vi "Get Named Range (String).vi"(8 "error in":errorcluster, 10 "Named Range Identifier":string, 11 "SpreadsheetDocument":refnum<k24>) -> (0 "error out":errorcluster, 2 "Cells":string[][](array[string]), 3 "SpreadsheetDocument out":refnum<k24>)   [LabVIEW 2021, in "Open Xml.lvlib"]
uses:
  Open Xml.lvlib
  C:/Users/tupp_js/.nuget/packages/documentformat.openxml/3.3.0/lib/net46/DocumentFormat.OpenXml.dll
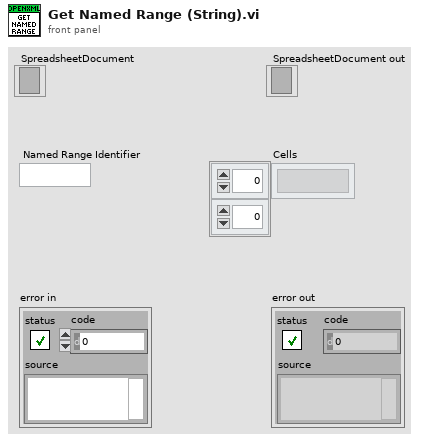
[diagram p1: front panel]
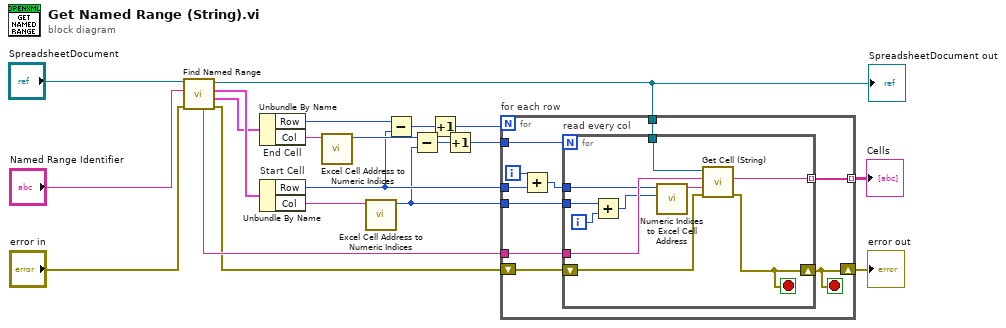
[diagram p0: block diagram]
diagram:
  n1 = call "Find Named Range.vi"("error in"="error in", "Range Identifier"="Named Range Identifier", "SpreadsheetDocument"="SpreadsheetDocument") -> ("error out"=w4:errorcluster, "End Cell"=w18:cluster{"Col":string, "Row":i32}, "Start Cell"=w19:cluster{"Col":string, "Row":i32}, "SpreadsheetDocument"=w1:refnum<k24>, "Sheet Name"=w6:string)  [unwired: 4 in]
  "SpreadsheetDocument out" <- w1
  n2 = Unbundle By Name "End Cell"(w18) -> ("Row"=w11:i32, "Col"=w16:string)
  n3 = Unbundle By Name "Start Cell"(w19) -> ("Row"=w8:i32, "Col"=w17:string)
  n4 = call "Excel Cell Address to Numeric Indices.vi"("Cell Name"=w16) -> ("Column Number"=w14:i32)  [unwired: 9 in, 1 out]
  n5 = call "Excel Cell Address to Numeric Indices.vi"("Cell Name"=w17) -> ("Column Number"=w7:i32)  [unwired: 9 in, 1 out]
  n6 = Subtract(x=w11, y=w8) -> (x-y=w10:i32)
  n7 = Subtract(x=w14, y=w7) -> (x-y=w12:i32)
  n8 = Increment(x=w10) -> (x+1=w9:i32)
  n9 = Increment(x=w12) -> (x+1=w13:i32)
  n10 = for "for each row" {
    N: w9 -> [_]
    tunnel: w13 -> [w30]
    tunnel: w8 -> [w26]
    tunnel: w1 -> [w29]
    tunnel: w7 -> [w28]
    tunnel: w6 -> [w27]
    tunnel: [w25] -> w5 mode=indexing
    shift-right: [w21] -> w3
    shift-left: w4 -> [w22]
    i -> [w23]
    stop <- w21 stop-if-true
    n11 = Add(x=w23, y=w26) -> (x+y=w24:i32)
    n12 = for "read every col" {
      N: w30 -> [_]
      tunnel: w29 -> [w40]
      tunnel: w28 -> [w37]
      tunnel: w27 -> [w39]
      tunnel: w24 -> [w36]
      tunnel: [w35] -> w25 mode=indexing
      shift-right: [w31] -> w21
      shift-left: w22 -> [w32]
      i -> [w33]
      stop <- w31 stop-if-true
      n13 = Add(x=w37, y=w33) -> (x+y=w34:i32)
      n14 = call "Numeric Indices to Excel Cell Address.vi"("Column"=w34, "Row"=w36) -> ("Cell Address"=w38:string)  [unwired: 9 in]
      n15 = call "Get Cell (String).vi"("error in"=w32, "Cell Address"=w38, "Sheet Name"=w39, "SpreadsheetDocument"=w40) -> ("error out"=w31:errorcluster, "Value String"=w35:string)  [unwired: 5 in, 1 out]
    }
  }
  "error out" <- w3
  "Cells" <- w5
